vi "Pick User.vi"(0 "User Manager View in":refnum<class "User Manager View.lvclass">, 5 "NewVal":i32, 11 "error in (no error)":errorcluster) -> (4 "User Manager View out":refnum<class "User Manager View.lvclass">, 15 "error out":errorcluster)   [LabVIEW 2017, in "User Manager View.lvlib" / "User Manager View.lvclass"]
uses:
  <vilib>/gpm_packages/@cs/User Manager App/User Manager View/User Manager View/User Manager View.lvclass
  <vilib>/gpm_packages/@cs/User Manager App/User Manager Model/Type Definitions/User Levels.ctl
  <vilib>/gpm_packages/@cs/User Manager App/User Manager View/User Manager View/User Manager View.lvclass/User Manager View.ctl
  <vilib>/gpm_packages/@cs/User Manager App/User Manager Model/Type Definitions/User Manager Application Types.lvlib
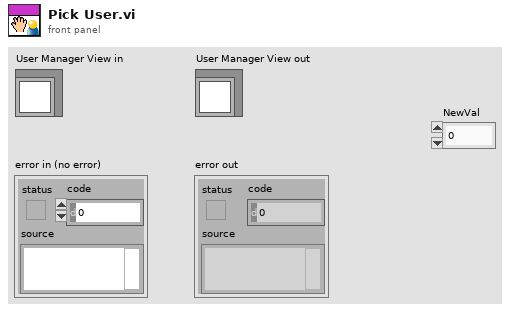
[diagram p1: front panel]
types:
  T1 = typedef "User Manager Application Types.lvlib/User Levels.ctl" = cluster{"Rank":i32, "Title":string}
  T2 = enum8{"Enabled", "Disabled", "Disabled and Grayed Out"}
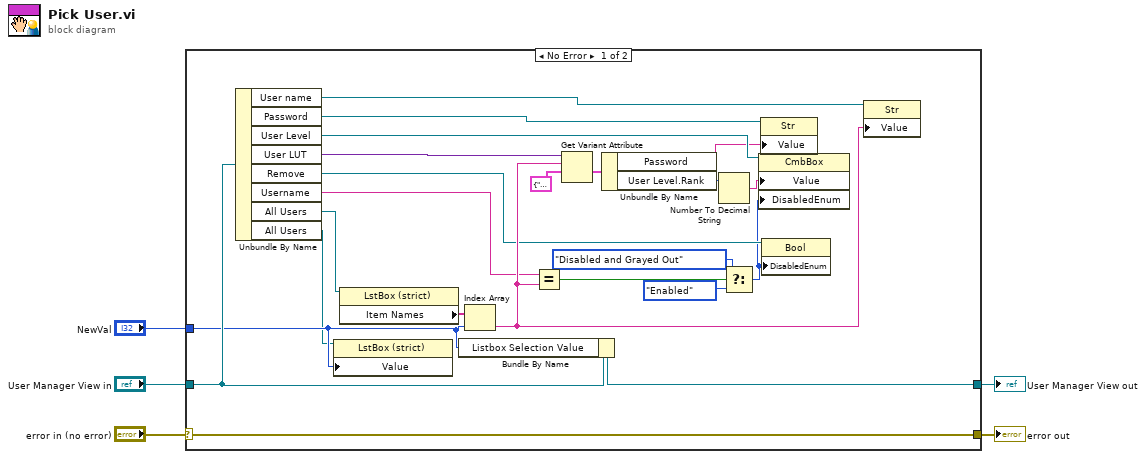
[diagram p0: block diagram]
diagram:
  n1 = case shown="No Error" "error in (no error)" {
    selector: "error in (no error)" -> [w28 w30]
    tunnel: [w28 w30] -> w4
    tunnel: [w16 w29] -> w2
    tunnel: "User Manager View in" -> [w27 w29]
    tunnel: "NewVal" -> [w8 _]
    frame No Error {
      n2 = Unbundle By Name(w27) -> ("User name"=w24:refnum<vi>, "Password"=w23:refnum<vi>, "User Level"=w22:refnum<vi>, "User LUT"=w14:variant, "Remove"=w12:refnum<vi>, "Username"=w11:string, "All Users"=w13:refnum<vi>, "All Users"=w7:refnum<vi>)
      n3 = property class="LstBox (strict)"(reference=w7, "Value"=w8) -> ()  [unwired: 1 in, 2 out]
      n4 = property class="LstBox (strict)"(reference=w13) -> ("Item Names"=w26:string[])  [unwired: 1 in, 2 out]
      n5 = Bundle By Name(cluster=w27, "Listbox Selection Value"=w8) -> (w16:refnum<class "User Manager View.lvclass">)
      n6 = Index Array(array=w26, index=w8) -> (element=w20:string)
      n7 = Equal?(x=w11, y=w20) -> (x = y?=w19:bool)
      n8 = Get Variant Attribute(Variant=w14, name=w20, default value (empty Variant)=cluster{"Password":string, "User Level":T1} {"Password"="", "User Level"={"Rank"=0, "Title"=""}}) -> (value=w25:cluster{"Password":string, "User Level":T1})  [unwired: 1 in, 3 out]
      n9 = Unbundle By Name(w25) -> ("Password"=w21:string, "User Level.Rank"=w10:i32)
      n10 = Number To Decimal String(number=w10) -> (decimal integer string=w9:string)  [unwired: 1 in]
      n11 = Select(t=T2."Disabled and Grayed Out", s=w19, f=T2."Enabled" ("Disabled")) -> (s? t:f=w6:T2)
      n12 = property class="CmbBox"(reference=w22, "Value"=w9, "DisabledEnum"=w6) -> ()  [unwired: 1 in, 2 out]
      n13 = property class="Str"(reference=w23, "Value"=w21) -> ()  [unwired: 1 in, 2 out]
      n14 = property class="Bool"(reference=w12, "DisabledEnum"=w6) -> ()  [unwired: 1 in, 2 out]
      n15 = property class="Str"(reference=w24, "Value"=w20) -> ()  [unwired: 1 in, 2 out]
    }
    frame Error {
    }
  }
  "error out" <- w4
  "User Manager View out" <- w2
